vi "Tray Icon Example.vi"() -> ()   [LabVIEW 2016]
doc: "Demonstrates the Tray Icon menu type. Run the VI to see the menu and icon appear in the system tray. Right click the icon to see the menu appear. Double click the Icon to signal a \"Default\" menu item click. Fill in the Balloon Info values and click \"Show Balloon\" to see the balloon pop-up in the system tray. The \"tipText\" is the only field required in the balloon info and an error will be thrown if you try to show a balloon with no tipText. the minimum timeout is controlled by the OS and any value less than the OS value will be coerced up\n\nClick summarys show up in the history array. Click the \"Add Item\" to add a dummy item to the TrayIcon's menu."
uses:
  <userlib>/_MGI/Menu Building/MenuTypes/TrayIcon/BalloonInfo.ctl
  <userlib>/_MGI/Menu Building/SelectionType/RadioSelection/MGI_RadioSelection.lvclass
  C:/Program Files (x86)/National Instruments/LabVIEW 2016/user.lib/_MGI/Menu Building/SelectionType/MGI_SelectionType.lvclass
  <userlib>/_MGI/Menu Building/SelectionType/CheckmarkSelection/MGI_CheckmarkSelection.lvclass
  <userlib>/_MGI/Menu Building/MenuItem/TrayIcon/MGI_TrayItem.lvclass
  C:/Program Files (x86)/National Instruments/LabVIEW 2016/user.lib/_MGI/Menu Building/MenuItem/MGI_MenuItem.lvclass
  <userlib>/_MGI/Menu Building/MenuItem/MenuSeparatorItem/MGI_MenuSeparatorItem.lvclass
  <userlib>/_MGI/Menu Building/MenuTypes/TrayIcon/MGI_TrayIcon.lvclass
  C:/Program Files (x86)/National Instruments/LabVIEW 2016/user.lib/_MGI/Menu Building/MenuTypes/MGI_Menu.lvclass
  <userlib>/_MGI/Menu Building/MenuItem/MenuItem.vi
  <userlib>/_MGI/Menu Building/SelectionType/RadioSelection/RadioSelection.vi
  <userlib>/_MGI/Menu Building/MenuItem/Write Click By Default.vi
  <userlib>/_MGI/Menu Building/MenuItem/Write Sub-Menus.vi
  <userlib>/_MGI/Menu Building/MenuTypes/TrayIcon/TrayIcon.vi
  <userlib>/_MGI/Menu Building/MenuItem/MenuSeparatorItem/MenuSeparatorItem.vi
  <userlib>/_MGI/Menu Building/SelectionType/CheckmarkSelection/CheckmarkSelection.vi
  <userlib>/_MGI/Menu Building/MenuItem/TrayIcon/TrayItem.vi
  <userlib>/_MGI/Menu Building/MenuItem/TrayIcon/Write DefaultItem.vi
  <userlib>/_MGI/Menu Building/MenuItem/Read Full Tag.vi
  <userlib>/_MGI/Menu Building/MenuTypes/Read Menu Items.vi
  <userlib>/_MGI/Menu Building/MenuItem/MGI_MenuItem.lvclass
  <userlib>/_MGI/Menu Building/MenuTypes/MGI_Menu.lvclass
  <userlib>/_MGI/Menu Building/SelectionType/MGI_SelectionType.lvclass
  <userlib>/_MGI/Menu Building/MenuItemStatusChange/MGI_MenuItemStatusChange.lvclass
panel:
  out "History":T1(array[cluster])
  in  "Add Item":bool
  in  "Show Balloon":bool
  in  "Balloon Info":T2
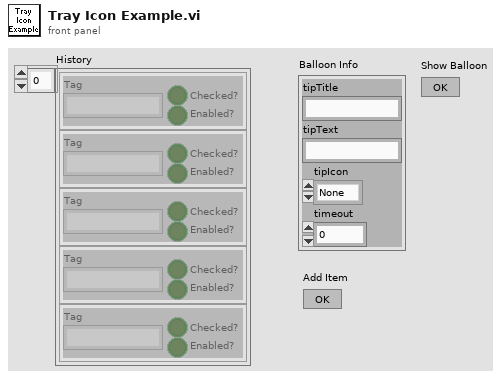
[diagram p1: front panel]
types:
  T1 = cluster{"Tag":string, "Checked?":bool, "Enabled?":bool}[]
  T2 = typedef "MGI_TrayIcon.lvclass/BalloonInfo.ctl" = cluster{"tipTitle":string, "tipText":string, "tipIcon":enum16{"None", "Info", "Warning", "Error"}, "timeout":i32}
  T3 = cluster{"Tag":string, "Checked?":bool, "Enabled?":bool}
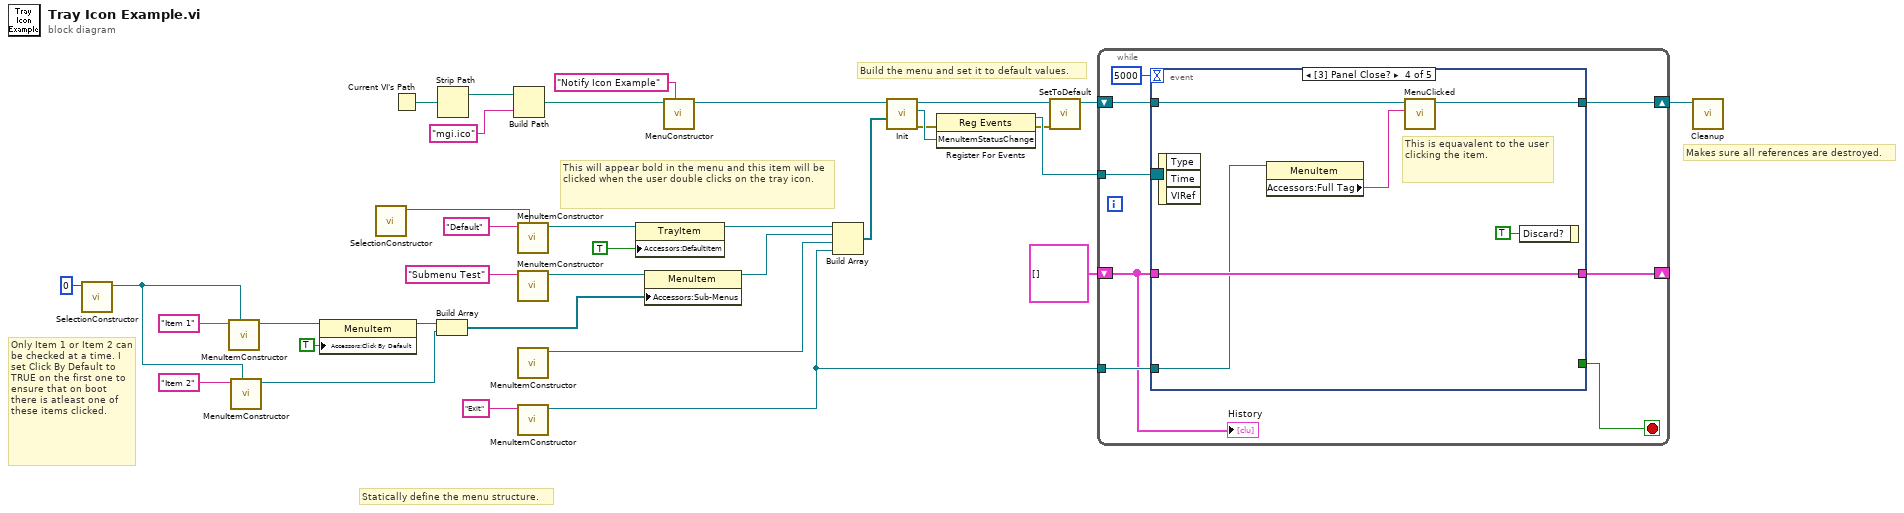
[diagram p0: block diagram]
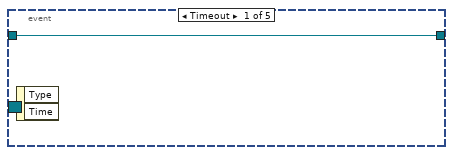
[diagram p2: hidden frame]
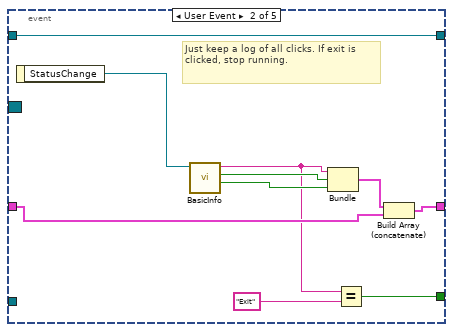
[diagram p3: hidden frame]
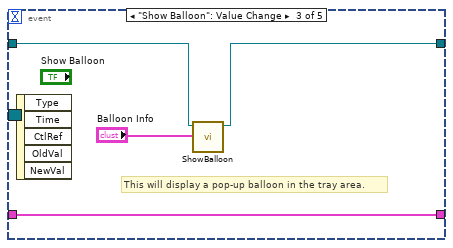
[diagram p4: hidden frame]
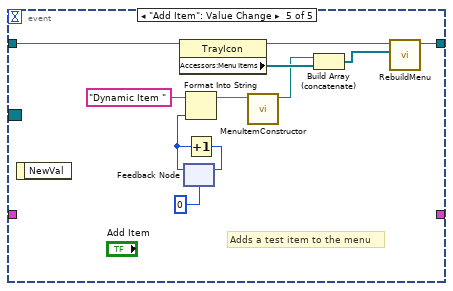
[diagram p5: hidden frame]
diagram:
  # "Makes sure all references are destroyed."
  # "Build the menu and set it to default values."
  # "This will appear bold in the menu and this item will be clicked when the user double clicks on the tray icon."
  # "Only Item 1 or Item 2 can be checked at a time. I set Click By Default to TRUE on the first one to ensure that on boot there is atleast one of these items clicked."
  # "Statically define the menu structure."
  n1 = call-poly <userlib>:"SelectionConstructor.vi"("Group"=u8 0) -> ("RadioSelection out"=w7:refnum<class "MGI_RadioSelection.lvclass">)  [unwired: 9 in, 1 out]
  n2 = call-poly <userlib>:"MenuItemConstructor.vi"("Selection Type"=w7, "Text"="Item 1") -> ("MenuItem"=w8:refnum<data-value>)  [unwired: 8 in, 1 out]
  n3 = call-poly <userlib>:"MenuItemConstructor.vi"("Selection Type"=w7, "Text"="Item 2") -> ("MenuItem"=w9:refnum<data-value>)  [unwired: 8 in, 1 out]
  n4 = property class="MenuItem"(reference=w8, "Accessors:Click By Default"=TRUE ("Click By Default")) -> (reference out=w4:refnum<data-value>)  [unwired: 1 in, 1 out]
  n5 = call-poly <userlib>:"SelectionConstructor.vi"() -> ("CheckmarkSelection out"=w16:refnum<class "MGI_CheckmarkSelection.lvclass">)  [unwired: 10 in, 1 out]
  n6 = Current VI's Path() -> (path=w25:path)
  n7 = Build Array(w4, w9) -> (w27:refnum<data-value>[])
  n8 = Strip Path(path=w25) -> (stripped path=w24:path)  [unwired: 1 out]
  n9 = Build Path(base path=w24, name or relative path="mgi.ico") -> (appended path=w20:path)
  n10 = call-poly <userlib>:"MenuItemConstructor.vi"("Selection Type"=w16, "Text"="Default") -> ("Notify Icon Item"=w17:refnum<data-value>)  [unwired: 8 in, 1 out]
  n11 = call-poly <userlib>:"MenuItemConstructor.vi"("Text"="Submenu Test") -> ("MenuItem"=w14:refnum<data-value>)  [unwired: 9 in, 1 out]
  n12 = call-poly <userlib>:"MenuItemConstructor.vi"() -> ("MenuSeparatorItem"=w12:refnum<data-value>)  [unwired: 10 in, 1 out]
  n13 = call-poly <userlib>:"MenuItemConstructor.vi"("Text"="Exit") -> ("MenuItem"=w5:refnum<data-value>)  [unwired: 9 in, 1 out]
  n14 = property class="TrayItem"(reference=w17, "Accessors:DefaultItem"=TRUE ("DefaultItem")) -> (reference out=w35:refnum<data-value>)  [unwired: 1 in, 1 out]
  n15 = property class="MenuItem"(reference=w14, "Accessors:Sub-Menus"=w27) -> (reference out=w26:refnum<data-value>)  [unwired: 1 in, 1 out]
  n16 = call-poly <userlib>:"MenuConstructor.vi"("Mouseover Text"="Notify Icon Example" ("Icon Text"), "Icon Path"=w20) -> ("NotifyIcon out"=w18:refnum<class "MGI_TrayIcon.lvclass">)  [unwired: 8 in, 1 out]
  n17 = Build Array(w35, w26, w12, w5) -> (w22:refnum<data-value>[])
  n18 = call-dynamic "Init.vi"("Menu Items"=w22, "Menu in"=w18) -> ("error out"=w21:errorcluster, "MenuItemStatusChange"=w34:refnum<user-event>, "Menu out"=w31:refnum<class "MGI_TrayIcon.lvclass">)  [unwired: 7 in]
  n19 = register-events(error in=w21, w34) -> (reference out=w33:refnum<event-registration>, error out=w29:errorcluster)  [unwired: 1 in]
  n20 = call-dynamic "SetToDefault.vi"("error in (no error)"=w29, "Menu in"=w31) -> ("Menu out"=w30:refnum<class "MGI_TrayIcon.lvclass">)  [unwired: 8 in, 1 out]
  n21 = while {
    tunnel: w33 -> [w43]
    shift-right: [w41] -> _
    shift-left: T1 [] -> [w36]
    shift-right: [w38] -> w32
    shift-left: w30 -> [w39]
    tunnel: w5 -> [w37]
    stop <- w42 stop-if-true
    n22 = event shown="[3] Panel Close?" {
      selector: w43 -> [_ _ _ _ _]
      dyn-events: _ -> [_ _ _ _ _]
      timeout: 5000 -> [_ _ _ _ _]
      tunnel: [_ w53 _ _ _] -> w42
      tunnel: [_ w52 w57 w63 _] -> w41
      tunnel: w36 -> [_ w51 w57 w63 _]
      tunnel: w39 -> [w44 w50 w56 w62 w75]
      tunnel: [w44 w50 w55 w61 w72] -> w38
      tunnel: w37 -> [_ _ _ w60 _]
      event Timeout {
        n23 = event-data() -> ()  [unwired: 1 in, 2 out]
      }
      event User Event {
        # "Just keep a log of all clicks. If exit is clicked, stop running."
        n24 = event-data() -> ("StatusChange"=w49:refnum<class "MGI_MenuItemStatusChange.lvclass">)  [unwired: 1 in]
        n25 = call <userlib>:"BasicInfo.vi"("MGI_MenuItemStatusChange in"=w49) -> ("Enabled?"=w47:bool, "Checked?"=w48:bool, "Tag"=w46:string)  [unwired: 7 in, 1 out]
        n26 = Bundle("Tag"=w46, "Checked?"=w48, "Enabled?"=w47) -> (w45:T3)  [unwired: 1 in]
        n27 = Equal?(x=w46, y="Exit") -> (x = y?=w53:bool)
        n28 = Build Array (concatenate)(w45, w51) -> (w52:T1)
      }
      event "Show Balloon": Value Change {
        # "This will display a pop-up balloon in the tray area."
        n29 = event-data() -> ()  [unwired: 1 in, 5 out]
        n30 = call <userlib>:"ShowBalloon.vi"("Balloon Info"="Balloon Info", "NotifyIcon in"=w56) -> ("NotifyIcon out"=w55:refnum<class "MGI_TrayIcon.lvclass">)  [unwired: 8 in, 1 out]
      }
      event Panel Close? {
        # "This is equavalent to the user clicking the item."
        n31 = event-data() -> ()  [unwired: 1 in, 3 out]
        n32 = property class="MenuItem"(reference=w60) -> ("Accessors:Full Tag"=w59:string)  [unwired: 1 in, 2 out]
        n33 = call-dynamic "MenuClicked.vi"("Full Tag"=w59, "Menu in"=w62) -> ("Menu out"=w61:refnum<class "MGI_TrayIcon.lvclass">)  [unwired: 8 in, 1 out]
        n34 = event-data("Discard?"=TRUE) -> ()  [unwired: 1 in, 1 out]
      }
      event "Add Item": Value Change {
        # "Adds a test item to the menu"
        n35 = event-data() -> ()  [unwired: 1 in, 1 out]
        n36 = property class="TrayIcon"(reference=w75) -> (reference out=w73:refnum<class "MGI_TrayIcon.lvclass">, "Accessors:Menu Items"=w71:refnum<data-value>[])  [unwired: 1 in, 1 out]
        n37 = feedback #1(0) -> (w66:i32)
        n38 = Format Into String(initial string="Dynamic Item " ("Text"), w66) -> (resulting string=w67:string)  [unwired: 2 in, 1 out]
        n39 = Increment(x=w66) -> (x+1=w65:i32)
        n40 = feedback-in #1(w65) -> ()
        n41 = call-poly <userlib>:"MenuItemConstructor.vi"("Text"=w67) -> ("MenuItem"=w70:refnum<data-value>)  [unwired: 9 in, 1 out]
        n42 = Build Array (concatenate)(w70, w71) -> (w74:refnum<data-value>[])
        n43 = call <userlib>:"RebuildMenu.vi"("New Menu Items"=w74, "Menu in"=w73) -> ("Menu out"=w72:refnum<class "MGI_TrayIcon.lvclass">)  [unwired: 8 in, 1 out]
      }
    }
    "History" <- w36
  }
  n44 = call-dynamic "Cleanup.vi"("MGI_TrayIcon in"=w32) -> ()  [unwired: 10 in, 1 out]
